vi "HART_Checksum.vi"(10 "message":u8[](array[numeric])) -> (2 "message + chk":u8[](array[numeric]), 3 "Checksum":u8)   [LabVIEW 2016]
doc: "If output string = \"Error\", the input string was not bytes"
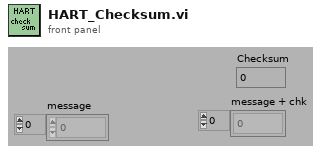
[diagram p1: front panel]
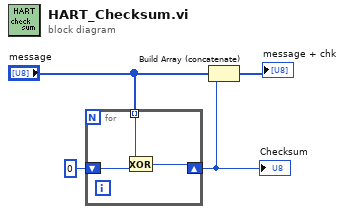
[diagram p0: block diagram]
diagram:
  n1 = for {
    shift-right: [w6] -> w2
    shift-left: u8 0 -> [w7]
    tunnel: "message" -> [w5] mode=indexing
    n2 = Exclusive Or(1:w7, 2:w5) -> (0:w6:u8)
  }
  "Checksum" <- w2
  n3 = Build Array (concatenate)("message", w2) -> (→"message + chk":u8[])
